vi "measuring loop time1.vi"() -> ()   [LabVIEW 2018]
panel:
  out "Loop iterations":i32
  in  "stop":bool
  in  "given loop time [ms]":i32=200
  out "measured loop time [ms]":u32
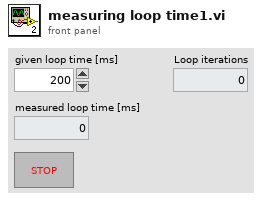
[diagram p1: front panel]
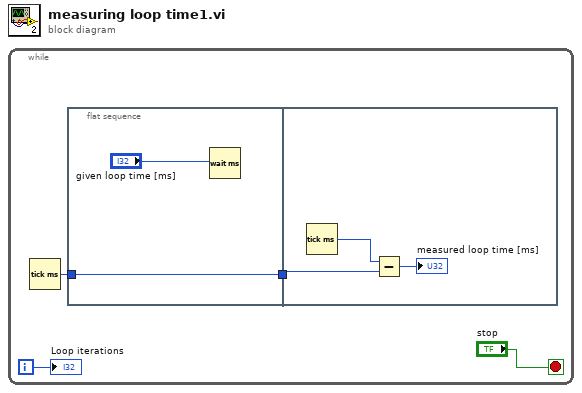
[diagram p0: block diagram]
diagram:
  n1 = while {
    i -> [w1]
    stop <- "stop" stop-if-true
    n2 = Tick Count (ms)() -> (millisecond timer value=w4:u32)
    n3 = flat-sequence {
      tunnel: w4 -> [w6]
      tunnel: [w6] -> w3
      tunnel: w3 -> [w7]
      frame #0 {
        n4 = Wait (ms)(milliseconds to wait="given loop time [ms]") -> ()  [unwired: 1 out]
      }
      frame #1 {
        n5 = Tick Count (ms)() -> (millisecond timer value=w8:u32)
        n6 = Subtract(x=w8, y=w7) -> (x-y=→"measured loop time [ms]":u32)
      }
    }
    "Loop iterations" <- w1
  }
